vi "reset.vi"(8 "error in (no error)":errorcluster, 11 "DL090430TriggeredExperimentController in":refnum<class "ExperimentControllerDL090803Triggered.lvclass">) -> (0 "error out":errorcluster, 3 "DL090430TriggeredExperimentController out":refnum<class "ExperimentControllerDL090803Triggered.lvclass">)   [LabVIEW 2010, in "ExperimentControllerDL090803Triggered.lvclass"]
uses:
  ExperimentControllerDL090803Triggered.lvclass
  ExperimentControllerDL090803Triggered.lvclass/ExperimentControllerDL090803Triggered.ctl
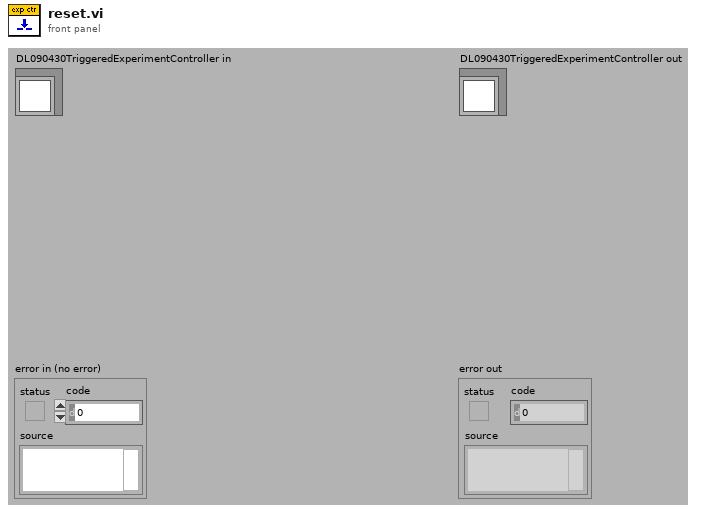
[diagram p1: front panel]
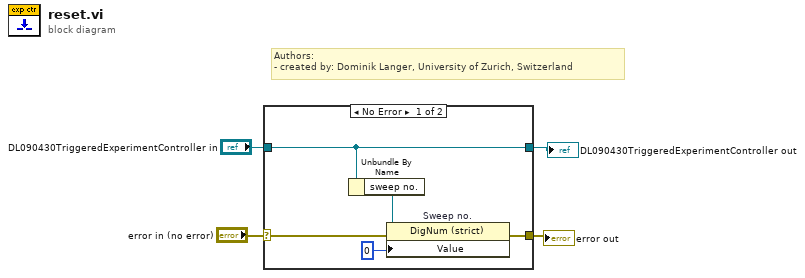
[diagram p0: block diagram]
diagram:
  # "Authors: \n- created by: Dominik Langer, University of Zurich, Switzerland"
  n1 = case shown="No Error" "error in (no error)" {
    selector: "error in (no error)" -> [w9 w11]
    tunnel: [w8 w11] -> w3
    tunnel: [w7 w10] -> w1
    tunnel: "DL090430TriggeredExperimentController in" -> [w7 w10]
    frame No Error {
      n2 = Unbundle By Name(w7) -> ("sweep no."=w6:refnum<vi>)
      n3 = property on="Sweep no." class="DigNum (strict)"(reference=w6, error in=w9, "Value"=0) -> (error out=w8:errorcluster)  [unwired: 1 out]
    }
    frame Error {
    }
  }
  "error out" <- w3
  "DL090430TriggeredExperimentController out" <- w1
